vi "testGetInstanceEvt.vi"(8 "error in (no error)":errorcluster) -> (0 "error out":errorcluster)   [LabVIEW 2018]
doc: "Test the getInstanceEvt.vi"
uses:
  src/TcpServer/TcpServer.lvclass
  src/TcpServerCmd/typedef/eventTypeDef.ctl
  src/TcpServerBase/typedef/tcpPacketTypeDef.ctl
  <vilib>/addons/_JKI Toolkits/Caraya/classes/Assert/Assert Equal Type_Variant.vi
  <vilib>/addons/_JKI Toolkits/Caraya/classes/Test/Test.lvclass
  <vilib>/addons/_JKI Toolkits/Caraya/classes/Assert/Assert.lvclass
  src/TcpServerCmd/TcpServerCmd.lvclass
  src/TcpServerBase/TcpServerBase.lvclass
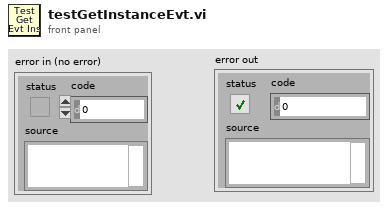
[diagram p1: front panel]
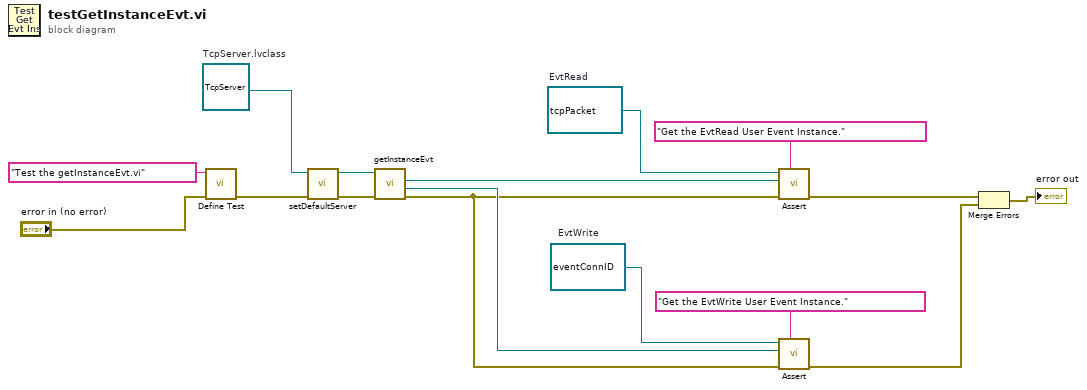
[diagram p0: block diagram]
diagram:
  w1 = refnum<user-event> refnum  # EvtRead
  w3 = refnum<user-event> refnum  # EvtWrite
  w13 = refnum<class "TcpServer.lvclass"> refnum  # TcpServer.lvclass
  n1 = call <vilib>:"Define Test.vi"("error in (no error)"="error in (no error)", "Label (VI Title)"="Test the getInstanceEvt.vi") -> ("error out"=w15:errorcluster)  [unwired: 9 in]
  n2 = call "setDefaultServer.vi"("error in (no error)"=w15, "TcpServer.lvclass"=w13) -> ("error out"=w10:errorcluster, "tcpServer out"=w11:refnum<class "TcpServer.lvclass">)  [unwired: 8 in]
  n3 = call "getInstanceEvt.vi"("error in (no error)"=w10, "tcpServer in"=w11) -> ("error out"=w2:errorcluster, "EvtWrite"=w4:refnum<user-event>, "EvtRead"=w9:refnum<user-event>)  [unwired: 6 in, 1 out]
  n4 = call-poly <vilib>:"Assert.vi"("Label"="Get the EvtRead User Event Instance.", "error in (no error)"=w2, "Y"=w9, "X"=w1) -> ("error out"=w8:errorcluster)  [unwired: 7 in]
  n5 = call-poly <vilib>:"Assert.vi"("Label"="Get the EvtWrite User Event Instance.", "error in (no error)"=w2, "Y"=w4, "X"=w3) -> ("error out"=w5:errorcluster)  [unwired: 7 in]
  n6 = Merge Errors(w8, w5) -> (→"error out":errorcluster)
